vi "Timer.vi"(8 "error in (no error)":errorcluster, 9 "Time Limit":dbl=5.0, 10 "Reset?":bool, 11 "Advance Time?":bool) -> (0 "error out":errorcluster, 2 "Time Elapsed":dbl=5.0, 3 "Time Expired?":bool)   [LabVIEW 2021]
doc: "Timer"
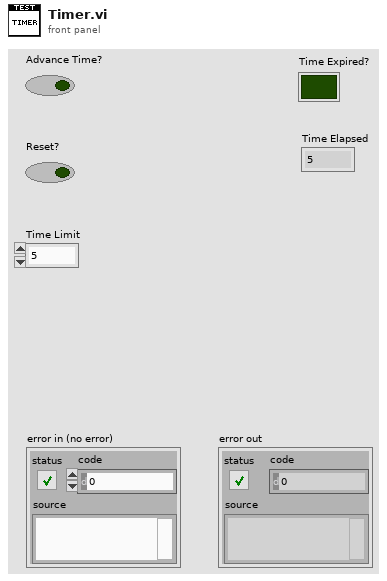
[diagram p1: front panel]
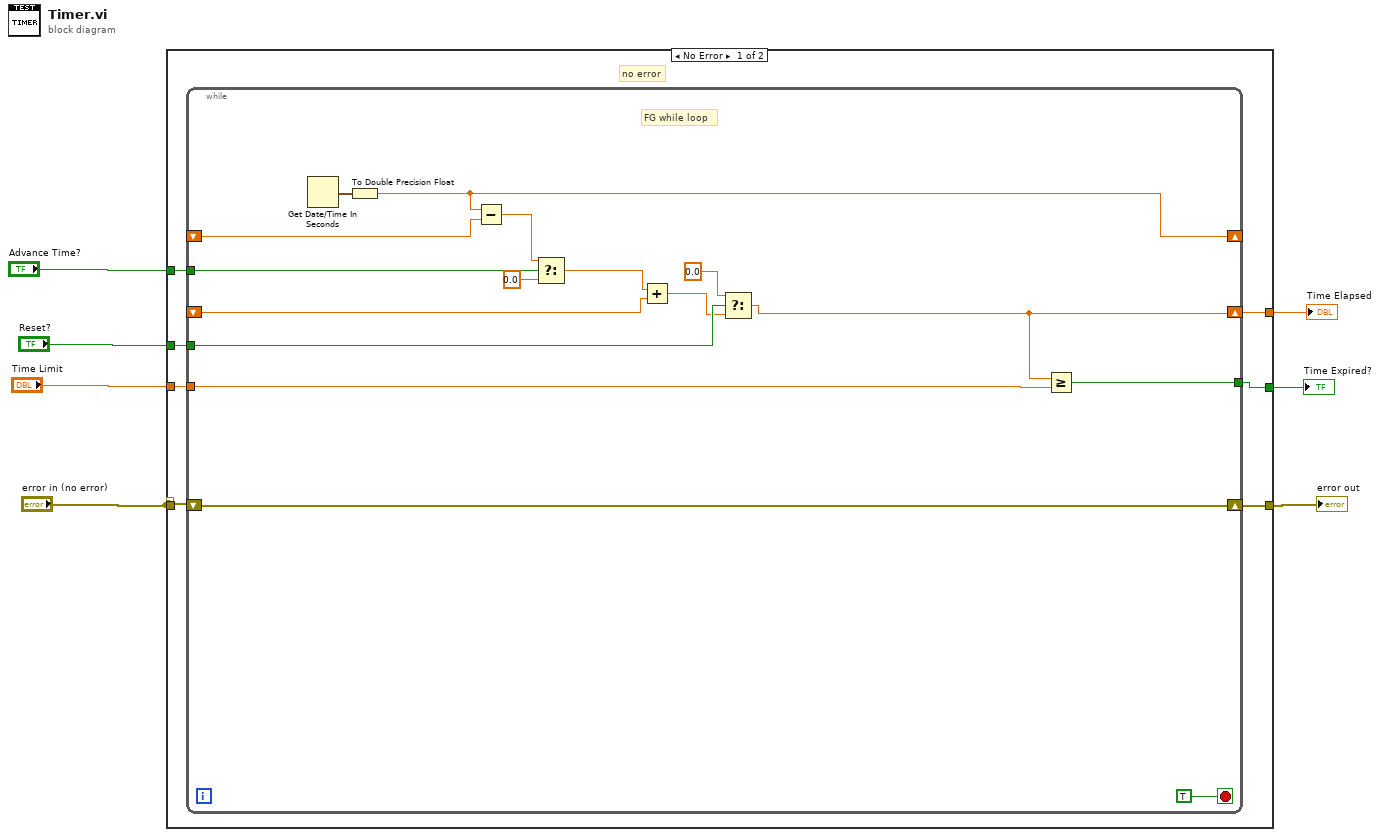
[diagram p0: block diagram]
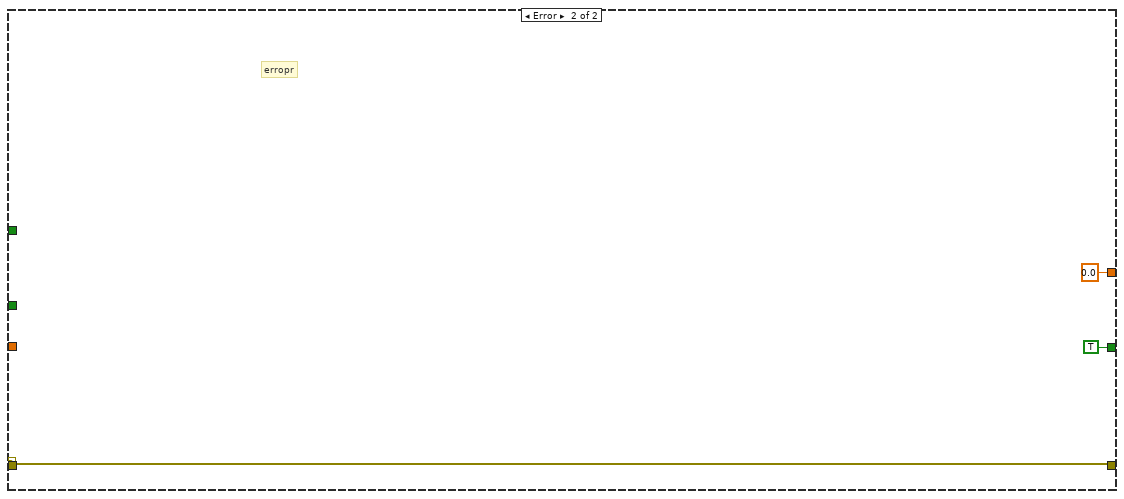
[diagram p2: hidden frame]
diagram:
  n1 = case shown="No Error" "error in (no error)" {
    selector: "error in (no error)" -> [w8 w31]
    tunnel: [w14 w31] -> w7
    tunnel: "error in (no error)" -> [_ _]
    tunnel: "Time Limit" -> [w13 _]
    tunnel: "Reset?" -> [w12 _]
    tunnel: "Advance Time?" -> [w11 _]
    tunnel: [w10 0.0 ("f")] -> w3
    tunnel: [w9 TRUE] -> w2
    frame No Error {
      # "no error"
      n2 = while {
        shift-right: [w30] -> w14
        shift-left: w8 -> [w30]
        tunnel: w13 -> [w20]
        tunnel: w12 -> [w21]
        tunnel: w11 -> [w24]
        shift-right: [w27] -> _
        shift-left: _ -> [w26]
        shift-right: [w19] -> w10
        shift-left: _ -> [w23]
        tunnel: [w18] -> w9
        stop <- TRUE stop-if-true
        # "FG while loop"
        n3 = Get Date/Time In Seconds() -> (seconds since 1Jan1904=w28:timestamp)
        n4 = To Double Precision Float(number=w28) -> (double precision float=w27:dbl)
        n5 = Subtract(x=w27, y=w26) -> (x-y=w25:dbl)
        n6 = Select(t=w25, s=w24, f=0.0) -> (s? t:f=w22:dbl)
        n7 = Add(x=w22, y=w23) -> (x+y=w16:dbl)
        n8 = Select(t=0.0 ("f"), s=w21, f=w16) -> (s? t:f=w19:dbl)
        n9 = Greater Or Equal?(x=w19, y=w20) -> (x >= y?=w18:bool)
      }
    }
    frame Error {
      # "erropr"
    }
  }
  "error out" <- w7
  "Time Expired?" <- w2
  "Time Elapsed" <- w3
